vi "Any_Char_Remove.vi"(2 "Individual Characters to Remove":string, 3 "String in":string) -> (0 "String out":string)   [LabVIEW 2012]
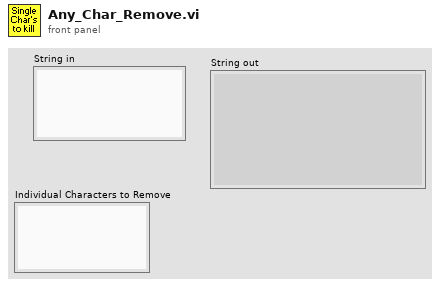
[diagram p1: front panel]
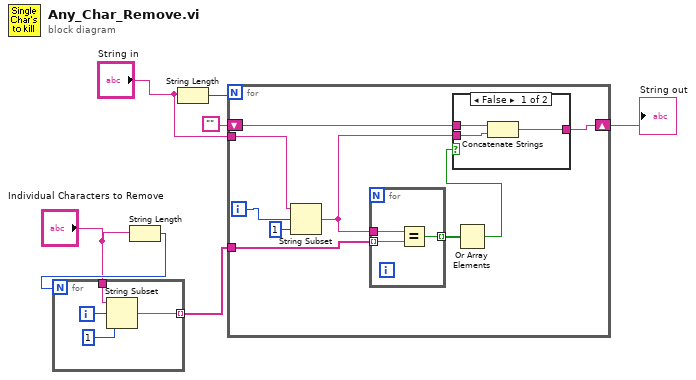
[diagram p0: block diagram]
diagram:
  n1 = String Length(string="Individual Characters to Remove") -> (length=w3:i32)
  n2 = for {
    N: w3 -> [_]
    tunnel: "Individual Characters to Remove" -> [w9]
    tunnel: [w8] -> w1 mode=indexing
    i -> [w11]
    n3 = String Subset(string=w9, offset (0)=w11, length (rest)=1 ("length (rest)")) -> (substring=w8:string)
  }
  n4 = String Length(string="String in") -> (length=w4:i32)
  n5 = for {
    N: w4 -> [_]
    tunnel: "String in" -> [w20]
    tunnel: w1 -> [w19]
    shift-right: [w17] -> w7
    shift-left: "" -> [w18]
    i -> [w16]
    n6 = String Subset(string=w20, offset (0)=w16, length (rest)=1 ("length (rest)")) -> (substring=w12:string)
    n7 = for {
      tunnel: w19 -> [w23] mode=indexing
      tunnel: w12 -> [w22]
      tunnel: [w21] -> w14 mode=indexing
      n8 = Equal?(x=w22, y=w23) -> (x = y?=w21:bool)
    }
    n9 = Or Array Elements(Boolean array=w14) -> (logical OR=w13:bool)
    n10 = case shown="False" w13 {
      tunnel: w18 -> [w26 w27]
      tunnel: [w25 w27] -> w17
      tunnel: w12 -> [w24 _]
      frame False {
        n11 = Concatenate Strings(w26, w24) -> (w25:string)
      }
      frame True {
      }
    }
  }
  "String out" <- w7
